vi "CalculateAmplitudeModulation.vi"(8 "input valid":bool=TRUE, 10 "AM_factor":fxp<+/-,16,2>, 11 "Data in":fxp<+/-,16,14>[](array[numeric])=[0.0, 0.0]) -> (0 "output valid":bool, 3 "Data out":fxp<+/-,16,14>[](array[numeric]))   [LabVIEW 2013]
doc: "Calculates various combinations on I_in, Q_in and cos(fi) and sin(fi) to be used later to delay the output signal"
uses:
  <vilib>/rvi/FXPMathLib/FxpInterpret/XNode/nifxpmath_Interpret.xnode
panel:
  in  "a_am":fxp<+/-,16,2>
  in  "b_am":fxp<+/-,16,2>
  in  "cos_am":fxp<+/-,16,0>
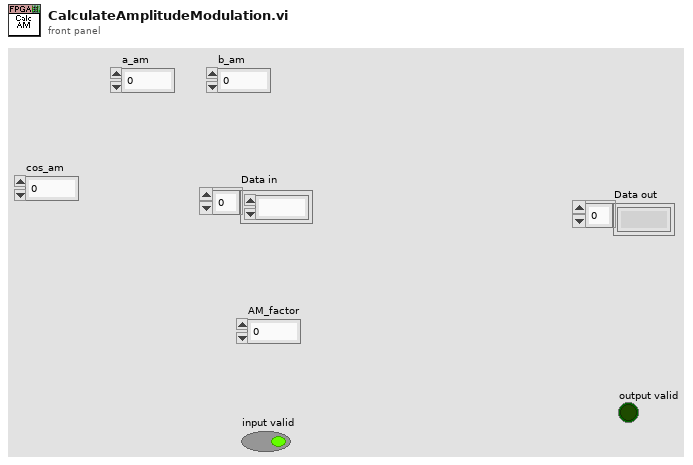
[diagram p1: front panel]
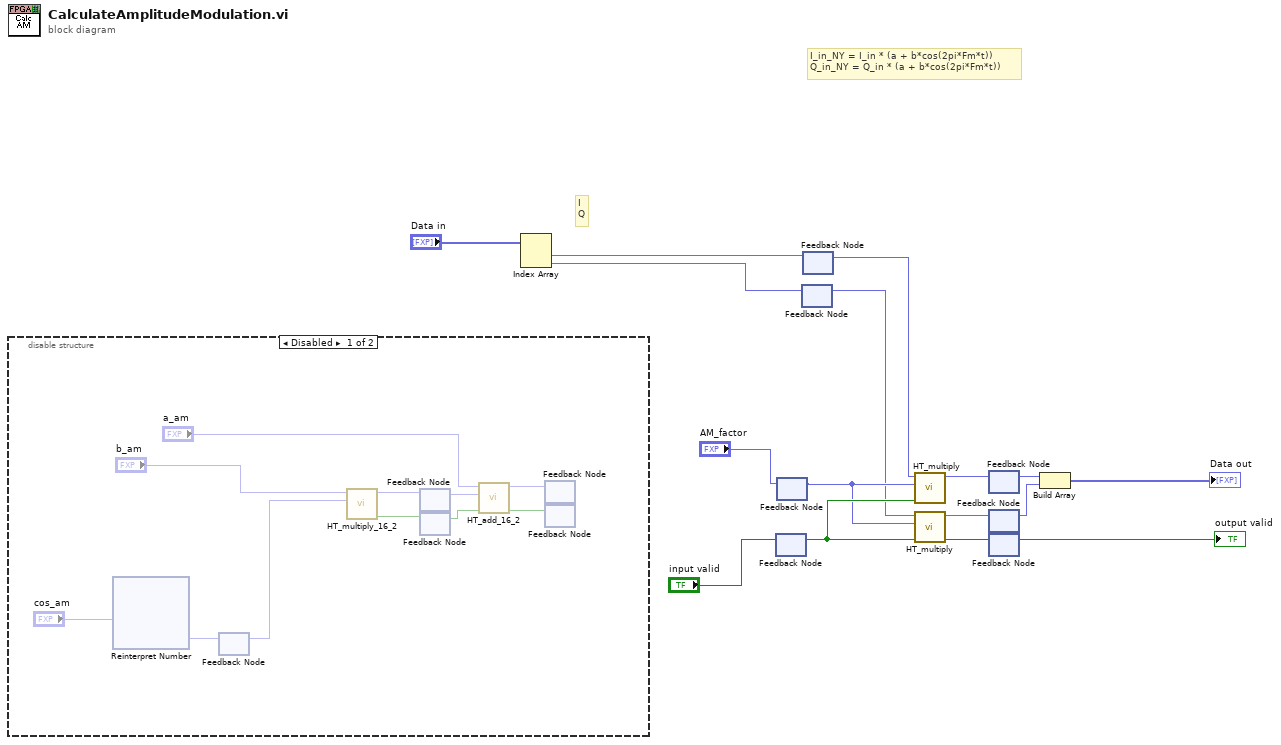
[diagram p0: block diagram]
diagram:
  # "I\nQ"
  # "I_in_NY = I_in * (a + b*cos(2pi*Fm*t))\nQ_in_NY = Q_in * (a + b*cos(2pi*Fm*t))"
  n1 = disable-structure shown="Disabled" {
    frame Disabled {
      n2 = xnode "Reinterpret Number"("x"="cos_am") -> ("y"=w27:fxp<+/-,16,2>)
      n3 = feedback #1() -> (w26:fxp<+/-,16,2>)  [unwired: 1 in]
      n4 = feedback-in #1(w27) -> ()
      n5 = call "HT_multiply_16_2.vi"("y"=w26, "x"="b_am") -> ("output valid"=w21:bool, "x*y"=w22:fxp<+/-,16,2>, "input valid"=w25:bool)  [unwired: 7 in]
      n6 = feedback #2() -> (w20:fxp<+/-,16,2>)  [unwired: 1 in]
      n7 = feedback-in #2(w22) -> ()
      n8 = feedback #3() -> (w19:bool)  [unwired: 1 in]
      n9 = feedback-in #3(w21) -> ()
      n10 = call "HT_add_16_2.vi"("input valid"=w19, "y"=w20, "x"="a_am") -> ("output valid"=w18:bool, "x+y"=w17:fxp<+/-,16,2>)  [unwired: 7 in]
      n11 = feedback #4() -> ()  [unwired: 2 in]
      n12 = feedback-in #4(w17) -> ()
      n13 = feedback #5() -> ()  [unwired: 2 in]
      n14 = feedback-in #5(w18) -> ()
    }
    frame Enabled {
    }
  }
  n15 = Index Array(array="Data in") -> (element #1=w4:fxp<+/-,16,14>, element #2=w2:fxp<+/-,16,14>)  [unwired: 2 in]
  n16 = feedback #6() -> (w7:bool)  [unwired: 1 in]
  n17 = feedback-in #6("input valid") -> ()
  n18 = feedback #7() -> (w5:fxp<+/-,16,2>)  [unwired: 1 in]
  n19 = feedback-in #7("AM_factor") -> ()
  n20 = feedback #8() -> (w1:fxp<+/-,16,14>)  [unwired: 1 in]
  n21 = feedback-in #8(w2) -> ()
  n22 = feedback #9() -> (w3:fxp<+/-,16,14>)  [unwired: 1 in]
  n23 = feedback-in #9(w4) -> ()
  n24 = call "HT_multiply.vi"("input valid"=w7, "y"=w5, "x"=w3) -> ("x*y"=w15:fxp<+/-,16,14>)  [unwired: 7 in, 1 out]
  n25 = call "HT_multiply.vi"("input valid"=w7, "y"=w5, "x"=w1) -> ("output valid"=w9:bool, "x*y"=w14:fxp<+/-,16,14>)  [unwired: 7 in]
  n26 = feedback #10() -> (w12:fxp<+/-,16,14>)  [unwired: 1 in]
  n27 = feedback-in #10(w15) -> ()
  n28 = feedback #11() -> (w11:fxp<+/-,16,14>)  [unwired: 1 in]
  n29 = feedback-in #11(w14) -> ()
  n30 = feedback #12() -> (→"output valid":bool)  [unwired: 1 in]
  n31 = feedback-in #12(w9) -> ()
  n32 = Build Array(w12, w11) -> (→"Data out":fxp<+/-,16,14>[])
